vi "Global 1.vi"() -> ()   [LabVIEW 2021]
panel:
  in  "mem":T1(c390)
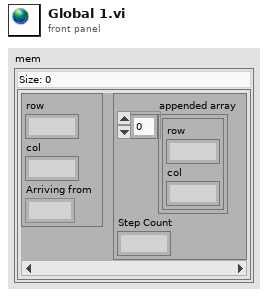
[diagram p1: front panel]
types:
  T1 = map{cluster{"row":i32, "col":i32, "Arriving from":enum16{"North", "South", "East", "West"}}, cluster{"appended array":cluster{"row":i32, "col":i32}[], "Step Count":u64}}
diagram:
